vi "_[error50002]Invalid DataType.vi"(8 "error in (no error)":errorcluster, 11 "string":string) -> (0 "error out":errorcluster)   [LabVIEW 2017, in "TagDB.lvlib"]
uses:
  TagDB.lvlib
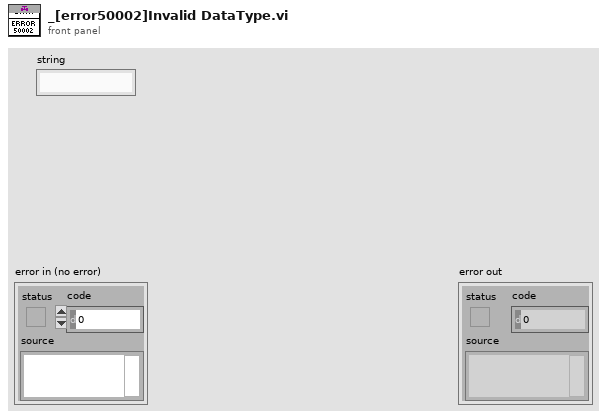
[diagram p1: front panel]
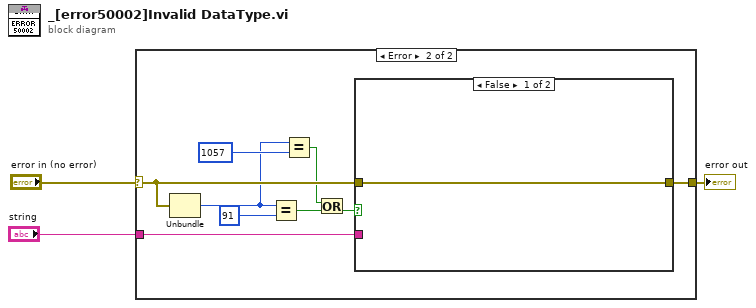
[diagram p0: block diagram]
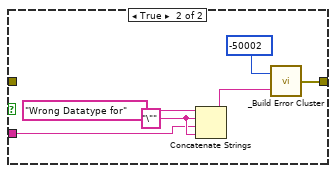
[diagram p3: hidden frame]
diagram:
  n1 = case shown="Error" "error in (no error)" {
    selector: "error in (no error)" -> [w4 w10]
    tunnel: [w4 w13] -> w3
    tunnel: "string" -> [_ w9]
    frame No Error {
    }
    frame Error {
      n2 = Unbundle(w10) -> ("code"=w6:i32)  [unwired: 2 out]
      n3 = Equal?(x=w6, y=91) -> (x = y?=w11:bool)
      n4 = Equal?(x=w6, y=1057) -> (x = y?=w5:bool)
      n5 = Or(x=w5, y=w11) -> (x .or. y?=w8:bool)
      n6 = case shown="False" w8 {
        tunnel: [w14 w16] -> w13
        tunnel: w10 -> [w14 _]
        tunnel: w9 -> [_ w18]
        frame False {
        }
        frame True {
          w19 = "\"" ("source")
          n7 = Concatenate Strings("Wrong Datatype for" ("source"), w19, w18, w19) -> (w17:string)
          n8 = call "_Build Error Cluster.vi"("String to Prepend to source (\"\")"=w17, "code"=-50002) -> ("error out"=w16:errorcluster)
        }
      }
    }
  }
  "error out" <- w3
